vi "Initialize.vi"(8 "error in (no error)":errorcluster, 10 "Path":path, 11 "FTPProtocol in":refnum<class "FTPProtocol.lvclass">) -> (0 "error out":errorcluster, 3 "FTPProtocol out":refnum<class "FTPProtocol.lvclass">)   [LabVIEW 2020, in "FileSync -- FTP.lvlib" / "FTPProtocol.lvclass"]
uses:
  FTPProtocol.lvclass
  FTPConfig/FTPConfig.lvclass
  _support/FTP Toolkit/FTP Class/FTP.lvclass
  FTPProtocol.lvclass/FTPProtocol.ctl
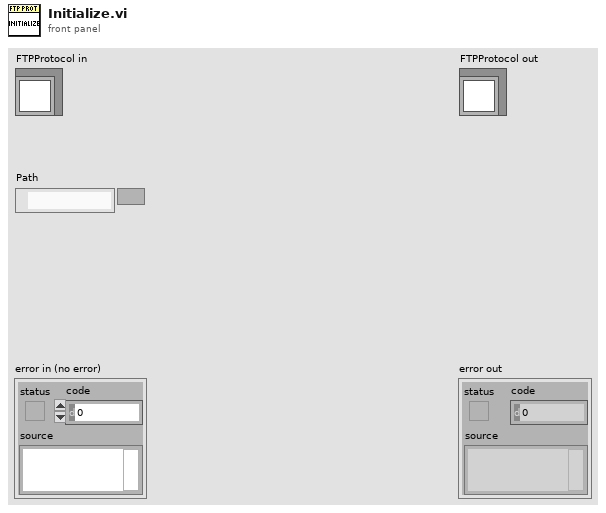
[diagram p1: front panel]
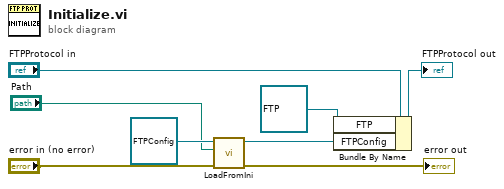
[diagram p0: block diagram]
diagram:
  n1 = call-dynamic "LoadFromIni.vi"("error in (no error)"="error in (no error)", "Path"="Path", "FTPConfig in"=refnum<class "FTPConfig.lvclass"> refnum ("FTPConfig")) -> ("error out"=→"error out":errorcluster, "FTPConfig out"=w2:refnum<class "FTPConfig.lvclass">)  [unwired: 7 in]
  n2 = Bundle By Name(cluster="FTPProtocol in", "FTP"=refnum<class "FTP.lvclass"> refnum, "FTPConfig"=w2) -> (→"FTPProtocol out":refnum<class "FTPProtocol.lvclass">)
